vi "Day 10 2D patterns.vi"() -> ()   [LabVIEW 2026]
panel:
  out "Array 3":string[][](array[string])
  out "Array 2":string[][](array[string])
  out "Array":string[][](array[string])
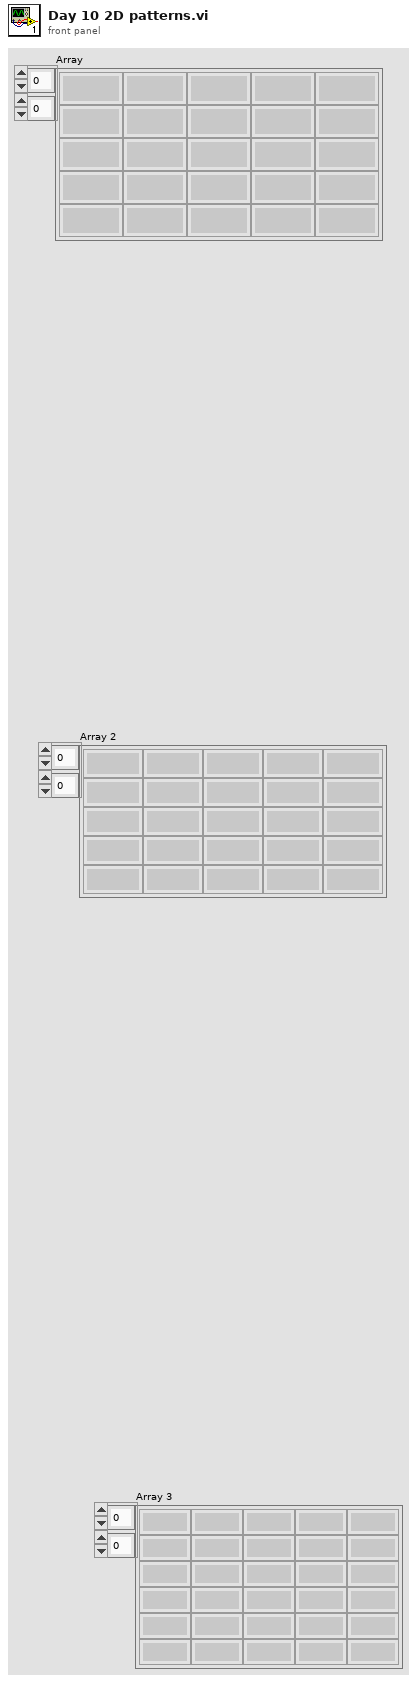
[diagram p1: front panel]
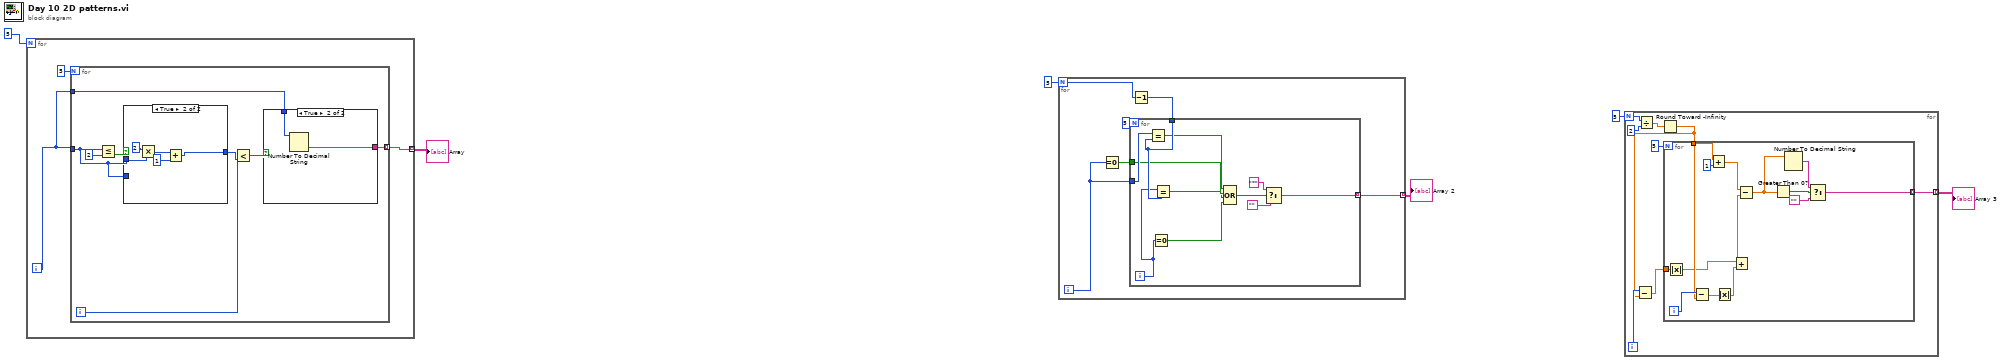
[diagram p0: block diagram]
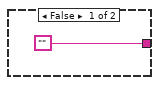
[diagram p2: hidden frame]
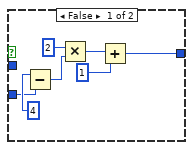
[diagram p3: hidden frame]
diagram:
  n1 = for {
    N: 5 -> [_]
    tunnel: [w7] -> w5 mode=indexing
    i -> [w8]
    n2 = for {
      N: 5 -> [_]
      tunnel: w8 -> [w15]
      tunnel: w8 -> [w13]
      tunnel: [w10] -> w7 mode=indexing
      i -> [w11]
      n3 = Less Or Equal?(x=w15, y=2) -> (x <= y?=w17:bool)
      n4 = case shown="True" w17 {
        tunnel: w15 -> [_ w31]
        tunnel: w15 -> [w25 _]
        tunnel: [w21 w28] -> w12
        frame False {
          n5 = Subtract(x=4, y=w25) -> (x-y=w24:i32)
          n6 = Multiply(x=2, y=w24) -> (x*y=w23:i32)
          n7 = Add(x=w23, y=1) -> (x+y=w21:i32)
        }
        frame True {
          n8 = Multiply(x=2, y=w31) -> (x*y=w30:i32)
          n9 = Add(x=w30, y=1) -> (x+y=w28:i32)
        }
      }
      n10 = Less?(x=w11, y=w12) -> (x < y?=w14:bool)
      n11 = case shown="True" w14 {
        tunnel: w13 -> [_ w20]
        tunnel: ["" w19] -> w10
        frame False {
        }
        frame True {
          n12 = Number To Decimal String(number=w20) -> (decimal integer string=w19:string)  [unwired: 1 in]
        }
      }
    }
  }
  "Array" <- w5
  n13 = for {
    N: 5 -> [w37]
    tunnel: [w33] -> w3 mode=indexing
    i -> [w36]
    n14 = Equal To 0?(x=w36) -> (x = 0?=w34:bool)
    n15 = Decrement(x=w37) -> (x-1=w35:i32)
    n16 = for {
      N: 5 -> [_]
      tunnel: w36 -> [w49]
      tunnel: w35 -> [w48]
      tunnel: w34 -> [w45]
      tunnel: [w39] -> w33 mode=indexing
      i -> [w47]
      n17 = Equal?(x=w49, y=w48) -> (x = y?=w46:bool)
      n18 = Equal To 0?(x=w47) -> (x = 0?=w43:bool)
      n19 = Equal?(x=w47, y=w48) -> (x = y?=w44:bool)
      n20 = Compound Arithmetic op=OR(w46, w45, w44, w43) -> (w42:bool)
      n21 = Select(t="*", s=w42, f="") -> (s? t:f=w39:string)
    }
  }
  "Array 2" <- w3
  n22 = for {
    N: 5 -> [w57]
    tunnel: [w50] -> w1 mode=indexing
    i -> [w54]
    n23 = Divide(x=w57, y=2) -> (x/y=w55:dbl)
    n24 = Round Toward -Infinity(1:w55) -> (0:w52:dbl)
    n25 = Subtract(x=w54, y=w52) -> (x-y=w51:dbl)
    n26 = for {
      N: 5 -> [_]
      tunnel: w52 -> [w69]
      tunnel: w51 -> [w65]
      tunnel: [w58] -> w50 mode=indexing
      i -> [w71]
      n27 = Absolute Value(x=w65) -> (abs(x)=w63:dbl)
      n28 = Subtract(x=w71, y=w69) -> (x-y=w70:dbl)
      n29 = Add(x=w69, y=1) -> (x+y=w67:dbl)
      n30 = Absolute Value(x=w70) -> (abs(x)=w64:dbl)
      n31 = Add(x=w63, y=w64) -> (x+y=w62:dbl)
      n32 = Subtract(x=w67, y=w62) -> (x-y=w61:dbl)
      n33 = Greater Than 0?(x=w61) -> (x > 0?=w66:bool)
      n34 = Number To Decimal String(number=w61) -> (decimal integer string=w60:string)  [unwired: 1 in]
      n35 = Select(t=w60, s=w66, f="") -> (s? t:f=w58:string)
    }
  }
  "Array 3" <- w1
